vi "IsVeriStandInstalled.vi"(8 "error in (no error)":errorcluster, 9 "Target IP Address":string, 10 "VS EXE Install Dir Uri":string, 11 "WebDav Ref In":T1) -> (0 "error out":errorcluster, 3 "WebDav Ref Out":T1)   [LabVIEW 2014]
doc: "Verifies that NI VeriStand is installed on the specified target"
uses:
  <vilib>/WebDAVClient/Advanced/SessionHandle.ctl
  <vilib>/Utility/error.llb/Error Cluster From Error Code.vi
  <vilib>/ErrorRing/Error Ring.xnode
  <vilib>/WebDAVClient/NI_WebDAV.lvlib
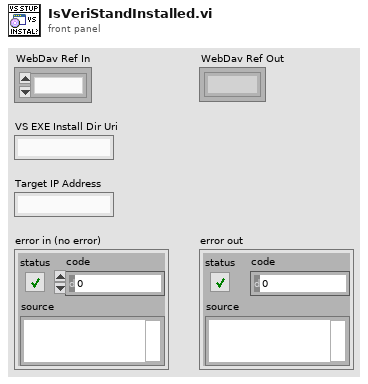
[diagram p1: front panel]
types:
  T1 = typedef "NI_WebDAV.lvlib/SessionHandle.ctl" = refnum<k1>
  T2 = typedef "NI_WebDAV.lvlib/FileInfo.ctl" = cluster{"type":string, "size":u64, "last modification":timestamp, "display name":string, "uri":string}
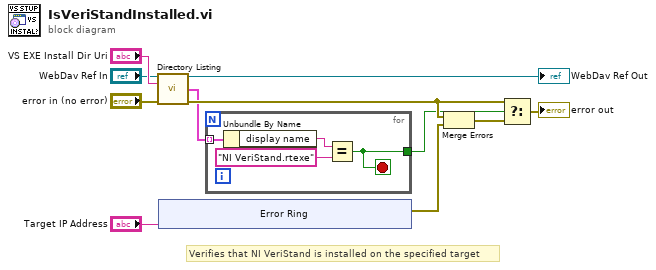
[diagram p0: block diagram]
diagram:
  # "Verifies that NI VeriStand is installed on the specified target"
  n1 = call <vilib>:"Directory Listing.vi"("session handle"="WebDav Ref In", "relative uri"="VS EXE Install Dir Uri", "error in (no error)"="error in (no error)") -> ("session handle out"=→"WebDav Ref Out":T1, "file list"=w4:T2[], "error out"=w10:errorcluster)  [unwired: 9 in, 1 out]
  n2 = xnode "Error Ring"("parameter 0"="Target IP Address") -> ("error out"=w11:errorcluster)
  n3 = for {
    tunnel: w4 -> [w15] mode=indexing
    tunnel: [w13] -> w5
    stop <- w13 stop-if-true
    n4 = Unbundle By Name(w15) -> ("display name"=w12:string)
    n5 = Equal?(x=w12, y="NI VeriStand.rtexe") -> (x = y?=w13:bool)
  }
  n6 = Merge Errors(w10, w11) -> (w9:errorcluster)
  n7 = Select(t=w10, s=w5, f=w9) -> (s? t:f=→"error out":errorcluster)
